vi "RandomSequence.vi"() -> ()   [LabVIEW 2017]
panel:
  out "Array":dbl[](array[numeric])
  out "nearest integer value":dbl
  in  "Numeric":i32
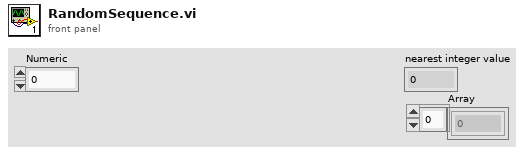
[diagram p1: front panel]
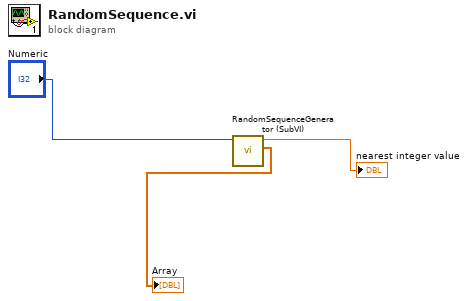
[diagram p0: block diagram]
diagram:
  n1 = call "RandomSequenceGenerator (SubVI).vi"("Numeric"="Numeric") -> ("Array"=→"Array":dbl[], "nearest integer value"=→"nearest integer value":dbl)  [unwired: 9 in]
